vi "REF_EDITOR_prepare_SELECT_statement.vi"(7 "nmb_of_top_rows (all)":i32, 8 "error_in":errorcluster) -> (0 "error_out":errorcluster, 3 "SELECT_statement":string)   [LabVIEW 2020]
uses:
  FGV/REF_EDITOR_records_display/FGV_REF_EDITOR_records_display.ctl
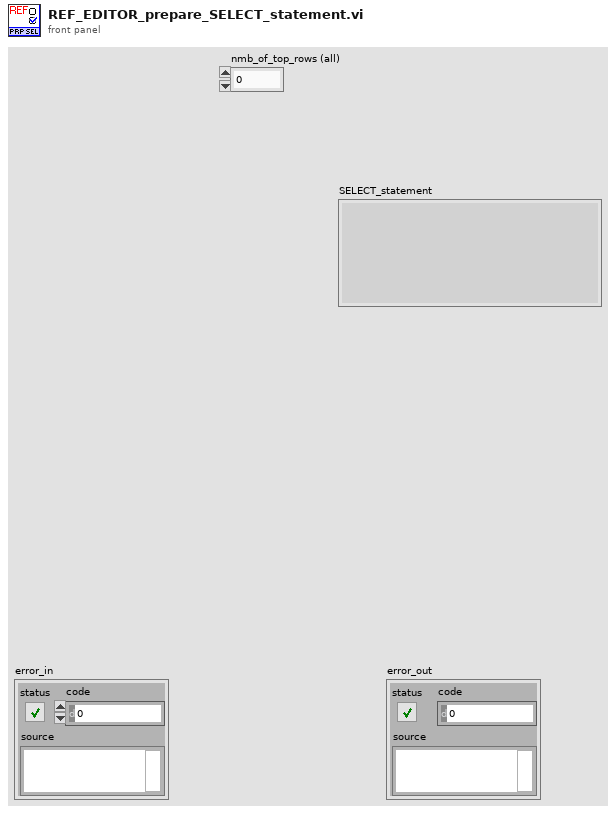
[diagram p1: front panel]
types:
  T1 = typedef "FGV_REF_EDITOR_records_display.ctl" = enum16{"initialize", "set_reference_tables_names", "set_station_number", "set_type_filter", "set_headers", "set_records", "set_reference_name", "change_actual_reference", "get_ref_table_name", "get_ref_hist_table_name", "get_station_number", "get_type_filter", "get_headers", "get_uneditable_columns", "get_all_info", "record_added?", "record_inserted?", "record_edited?", "record_updated?", "record_deleted?", "discard_changes"}
  T2 = typedef "REF_EDITOR_all_info.ctl" = cluster{"station_number":string, "type_filter":string, "reference_table":string, "reference_history":string, "headers":string[], "uneditable_columns":string[], "uneditable_columns":i32[], "editable_columns":i32[], "values_in_database":string[][], "size":cluster{"columns":i32, "SQL_rows":i32, "disp_rows":i32}, "REF_record_states":T3[], "actual_reference_name":string}
  T3 = typedef "SQL_record_states.ctl" = enum16{"Equal", "Added", "Edited", "Deleted"}
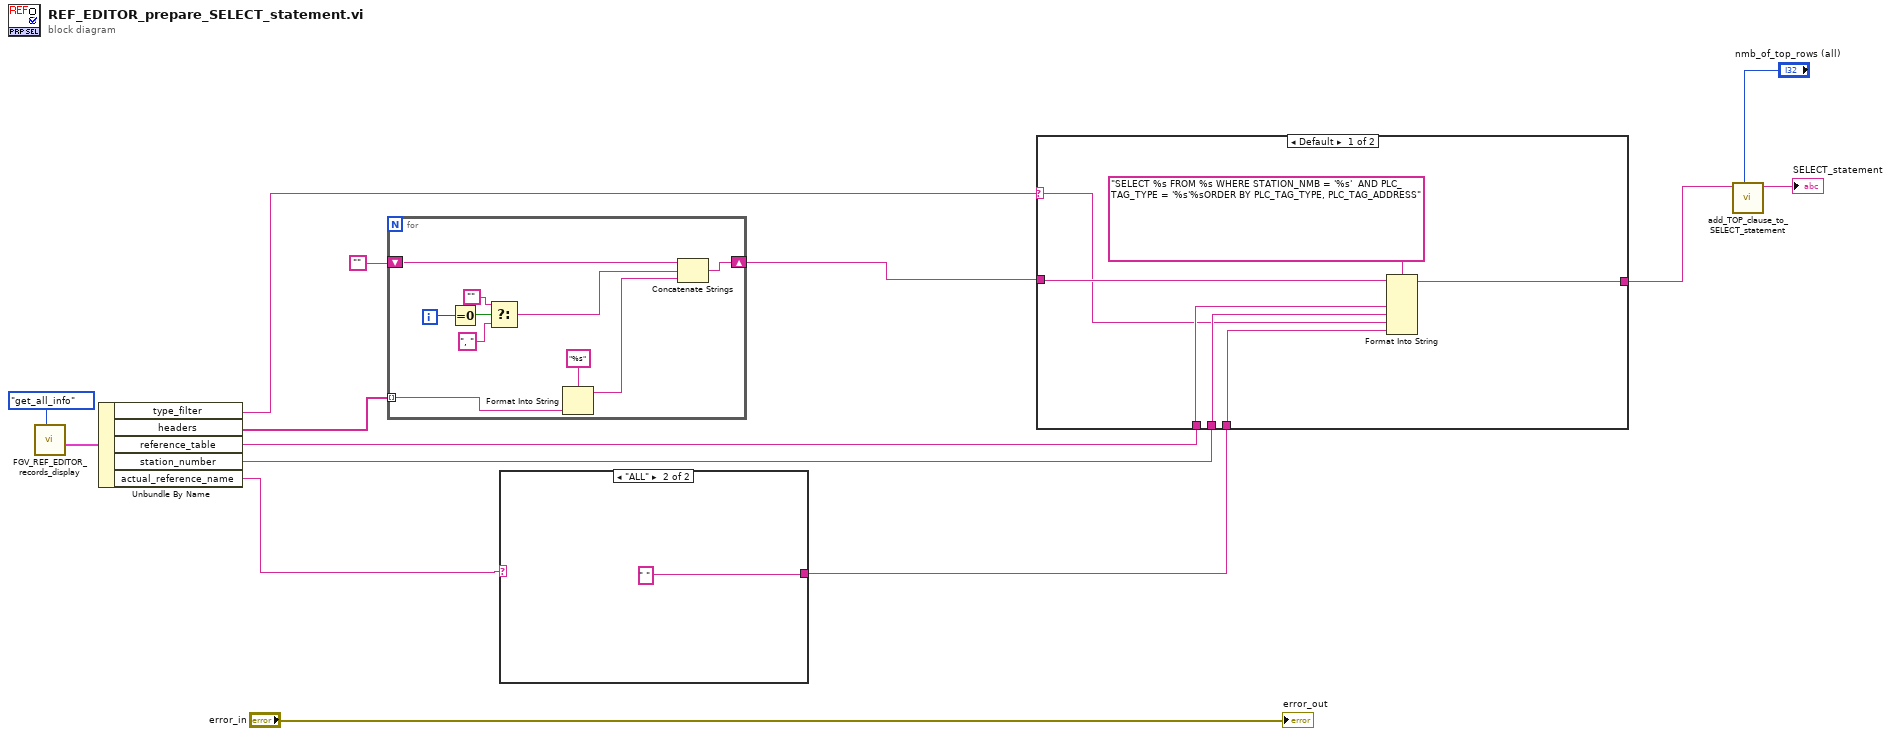
[diagram p0: block diagram]
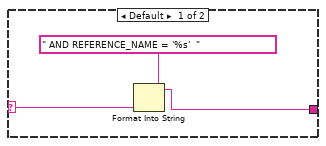
[diagram p2: hidden frame]
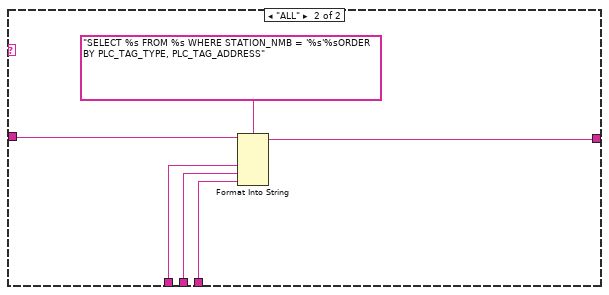
[diagram p3: hidden frame]
diagram:
  n1 = call "FGV_REF_EDITOR_records_display.vi"("options"=FGV_REF_EDITOR_records_display."get_all_info") -> ("all_info"=w4:T2)  [unwired: 7 in, 3 out]
  n2 = Unbundle By Name(w4) -> ("type_filter"=w3:string, "headers"=w11:string[], "reference_table"=w8:string, "station_number"=w7:string, "actual_reference_name"=w2:string)
  n3 = for {
    tunnel: w11 -> [w17] mode=indexing
    shift-right: [w19] -> w9
    shift-left: "" -> [w20]
    i -> [w24]
    n4 = Equal To 0?(x=w24) -> (x = 0?=w23:bool)
    n5 = Select(t="", s=w23, f=", ") -> (s? t:f=w18:string)
    n6 = Format Into String(format string="%s", w17) -> (resulting string=w16:string)  [unwired: 2 in, 1 out]
    n7 = Concatenate Strings(w20, w18, w16) -> (w19:string)
  }
  n8 = case shown="\"ALL\"" w2 {
    selector: w2 -> [w26 _]
    tunnel: [w25 " "] -> w1
    frame Default {
      n9 = Format Into String(format string=" AND REFERENCE_NAME = '%s'  ", w26) -> (resulting string=w25:string)  [unwired: 2 in, 1 out]
    }
    frame "ALL" {
    }
  }
  n10 = case shown="Default" w3 {
    selector: w3 -> [w30 _]
    tunnel: w9 -> [w34 w40]
    tunnel: w8 -> [w32 w39]
    tunnel: w7 -> [w31 w38]
    tunnel: [w33 w37] -> w6
    tunnel: w1 -> [w29 w36]
    frame Default {
      n11 = Format Into String(format string="SELECT %s FROM %s WHERE STATION_NMB = '%s'  AND PLC_TAG_TYPE = '%s'%sORDER BY PLC_TAG_TYPE, PLC_TAG_ADDRESS", w34, w32, w31, w30, w29) -> (resulting string=w33:string)  [unwired: 2 in, 1 out]
    }
    frame "ALL" {
      n12 = Format Into String(format string="SELECT %s FROM %s WHERE STATION_NMB = '%s'%sORDER BY PLC_TAG_TYPE, PLC_TAG_ADDRESS", w40, w39, w38, w36) -> (resulting string=w37:string)  [unwired: 2 in, 1 out]
    }
  }
  n13 = call "add_TOP_clause_to_SELECT_statement.vi"("nmb_of_top_rows (all)"="nmb_of_top_rows (all)", "SELECT_statement_in"=w6) -> ("SELECT_statement_out"=→"SELECT_statement":string)  [unwired: 8 in, 1 out]
  "error_out" <- "error_in"
